vi "get_max_interval.vi"(8 "error in (no error)":errorcluster, 11 "DAQmxWriteSignals in":refnum<class "SignalWriterDL090202DAQmx.lvclass">) -> (0 "error out":errorcluster, 1 "max value":dbl, 2 "min value":dbl, 3 "DAQmxWriteSignals out":refnum<class "SignalWriterDL090202DAQmx.lvclass">)   [LabVIEW 2010, in "SignalWriterDL090202DAQmx.lvclass"]
uses:
  SignalWriterDL090202DAQmx.lvclass
  C:/Program Files (x86)/National Instruments/LabVIEW 2010/resource/objmgr/daqmx.rc
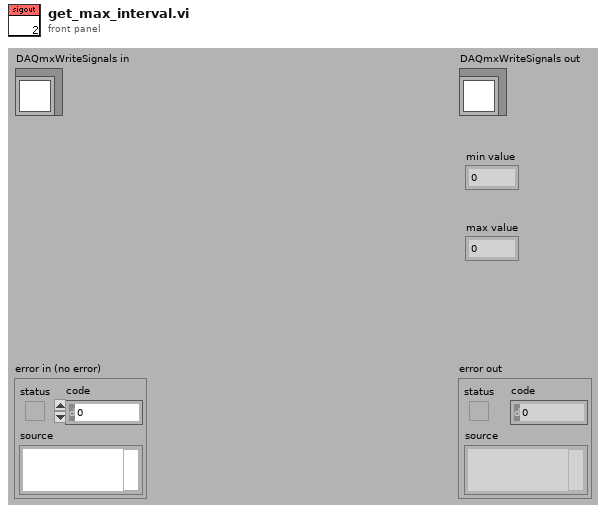
[diagram p1: front panel]
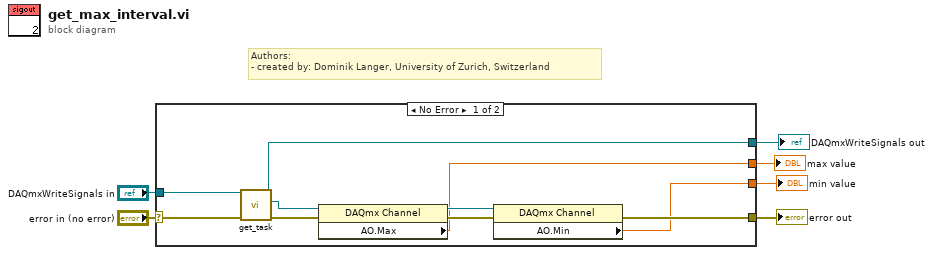
[diagram p0: block diagram]
diagram:
  # "Authors: \n- created by: Dominik Langer, University of Zurich, Switzerland"
  n1 = case shown="No Error" "error in (no error)" {
    selector: "error in (no error)" -> [w10 w18]
    tunnel: [w9 w18] -> w5
    tunnel: [w11 w17] -> w3
    tunnel: "DAQmxWriteSignals in" -> [w12 w17]
    tunnel: [w8 _] -> w2
    tunnel: [w7 _] -> w1
    frame No Error {
      n2 = call-dynamic "get_task.vi"("error in (no error)"=w10, "DAQmxWriteSignals in"=w12) -> ("error out"=w14:errorcluster, "writer task"=w16:refnum<k21>, "DAQmxWriteSignals out"=w11:refnum<class "SignalWriterDL090202DAQmx.lvclass">)  [unwired: 7 out]
      n3 = property class="DAQmx Channel"(reference=w16, error in=w14) -> (reference out=w13:refnum<k21>, error out=w15:errorcluster, "AO.Max"=w7:dbl)
      n4 = property class="DAQmx Channel"(reference=w13, error in=w15) -> (error out=w9:errorcluster, "AO.Min"=w8:dbl)  [unwired: 1 out]
    }
    frame Error {
    }
  }
  "error out" <- w5
  "DAQmxWriteSignals out" <- w3
  "min value" <- w2
  "max value" <- w1
